vi "StringToVarData.vi"(8 "error in (no error)":errorcluster, 10 "String Value":string, 11 "Variant ref":variant) -> (0 "error out":errorcluster, 3 "Varaint Out":variant)   [LabVIEW 2014, in "TableLogger_Actor.lvlib" / "TableLogger_Actor.lvclass"]
uses:
  TableLogger_Actor.lvclass
panel:
  # "Connector Pane"
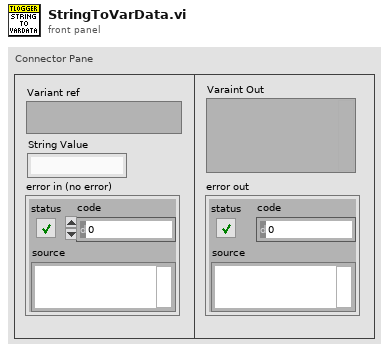
[diagram p1: front panel]
types:
  T1 = typedef "Type Descriptor Enumeration__ogtk.ctl" = enum8{"<Null>", "I8", "I16", "I32", "I64", "U8", "U16", "U32", "U64", "SGL", "DBL", "EXT", "CSG", "CDB", "CXT", "0x0F", "0x10", "0x11", "0x12", "0x13", "0x14", "Enum U8", "Enum U16", "Enum U32", "Enum U64", "SGL PQ", "DBL PQ", "EXT PQ", "CSG PQ", "CDB PQ", "CXT PQ", "0x1F", "0x20", "Boolean", "0x22", "0x23", "0x24", "0x25", "0x26", "0x27", "0x28", "0x29", "0x2A", "0x2B", "0x2C", "0x2D", "0x2E", "0x2F", "String", "0x31", "Path", "Pict", "0x34", "0x35", "0x36", "DAQ", "0x38", "0x39", "0x3A", "0x3B", "0x3C", "0x3D", "0x3E", "0x3F", "Array", "0x41", "0x42", "0x43", "0x44", "0x45", "0x46", "0x47", "0x48", "0x49", "0x4A", "0x4B", "0x4C", "0x4D", "0x4E", "0x4F", "Cluster", "0x51", "0x52", "Variant", "Waveform", "0x55", "0x56", "0x57", "0x58", "0x59", "0x5A", "0x5B", "0x5C", "0x5D", "0x5E", "0x5F", "0x60", "0x61", "0x62", "0x63", "0x64", "0x65", "0x66", "0x67", "0x68", "0x69", "0x6A", "0x6B", "0x6C", "0x6D", "0x6E", "0x6F", "Refnum"}
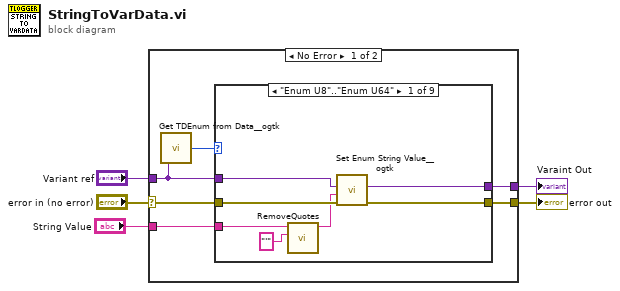
[diagram p0: block diagram]
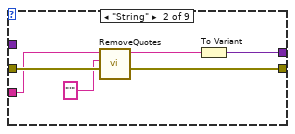
[diagram p2: hidden frame]
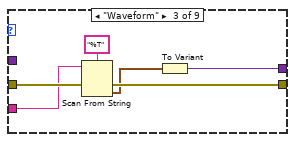
[diagram p3: hidden frame]
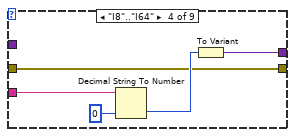
[diagram p4: hidden frame]
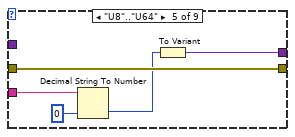
[diagram p5: hidden frame]
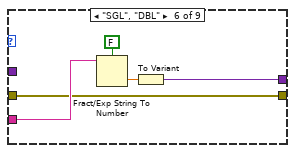
[diagram p6: hidden frame]
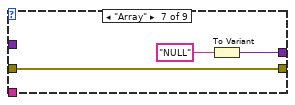
[diagram p7: hidden frame]
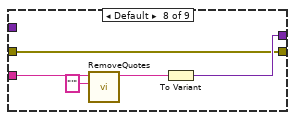
[diagram p8: hidden frame]
diagram:
  n1 = case shown="No Error" "error in (no error)" {
    selector: "error in (no error)" -> [w10 w54]
    tunnel: [w11 w54] -> w5
    tunnel: "Variant ref" -> [w9 _]
    tunnel: "String Value" -> [w7 _]
    tunnel: [w6 _] -> w1
    frame No Error {
      n2 = call <userlib>:"Get TDEnum from Data__ogtk.vi"("Data"=w9) -> ("Type Descriptor Enumeration"=w8:T1)  [unwired: 4 in]
      n3 = case shown="\"Enum U8\"..\"Enum U64\"" w8 {
        tunnel: w10 -> [w18 w22 w28 w30 w39 w40 w47 w51 w53]
        tunnel: w9 -> [w14 _ _ _ _ _ _ _ _]
        tunnel: [w15 w22 w27 w30 w39 w40 w47 w51 w53] -> w11
        tunnel: w7 -> [w16 w20 w26 w34 w36 w42 _ w50 _]
        tunnel: [w13 w23 w24 w31 w35 w41 w45 w52 _] -> w6
        frame "Enum U8".."Enum U64" {
          n4 = call "RemoveQuotes.vi"("replace string (\"\")"="'" ("replace string (\"\")"), "Input String in"=w16) -> ("Input String out"=w12:string)  [unwired: 9 in]
          n5 = call <userlib>:"Set Enum String Value__ogtk.vi"("error in (no error)"=w18, "String Value"=w12, "Default Enum Value"=w14) -> ("error out"=w15:errorcluster, "Enum"=w13:variant)  [unwired: 7 in]
        }
        frame "String" {
          n6 = call "RemoveQuotes.vi"("replace string (\"\")"="'" ("replace string (\"\")"), "Input String in"=w20) -> ("Input String out"=w19:string)  [unwired: 9 in]
          n7 = To Variant(anything=w19) -> (Variant=w23:variant)
        }
        frame "Waveform" {
          n8 = Scan From String(format string="%T", input string=w26, error in=w28) -> (error out=w27:errorcluster, output 1=w25:timestamp)  [unwired: 2 in, 2 out]
          n9 = To Variant(anything=w25) -> (Variant=w24:variant)
        }
        frame "I8".."I64" {
          n10 = Decimal String To Number(string=w34, default (0L)=i64 0) -> (number=w32:i64)  [unwired: 1 in, 1 out]
          n11 = To Variant(anything=w32) -> (Variant=w31:variant)
        }
        frame "U8".."U64" {
          n12 = Decimal String To Number(string=w36, default (0L)=i64 0) -> (number=w37:i64)  [unwired: 1 in, 1 out]
          n13 = To Variant(anything=w37) -> (Variant=w35:variant)
        }
        frame "SGL", "DBL" {
          n14 = Fract/Exp String To Number(use system decimal point (T)=FALSE, string=w42) -> (number=w44:dbl)  [unwired: 2 in, 1 out]
          n15 = To Variant(anything=w44) -> (Variant=w41:variant)
        }
        frame "Array" {
          n16 = To Variant(anything="NULL" ("String Value")) -> (Variant=w45:variant)
        }
        frame Default {
          n17 = call "RemoveQuotes.vi"("replace string (\"\")"="'" ("replace string (\"\")"), "Input String in"=w50) -> ("Input String out"=w49:string)  [unwired: 9 in]
          n18 = To Variant(anything=w49) -> (Variant=w52:variant)
        }
        frame "Cluster" {
        }
      }
    }
    frame Error {
    }
  }
  "error out" <- w5
  "Varaint Out" <- w1
